vi "Get Required Driver Type.vi"(8 "error in (no error)":errorcluster, 11 "DMM Msg in":refnum<class "DMM Msg.lvclass">) -> (0 "error out":errorcluster, 2 "Required Driver Type":refnum<class "Instrument Driver.lvclass">, 3 "DMM Msg out":refnum<class "DMM Msg.lvclass">)   [LabVIEW 2020, in "DMM Msg.lvlib" / "DMM Msg.lvclass"]
doc: "Get the Required Driver Type for execution of the Instrument Msg."
uses:
  DMM Msg.lvclass
  PPL/HDH.Actor Framework.Core.Instrument Driver.lvlibp/Instrument Driver/Instrument Driver.lvclass
  PPL/HDH.Driver.DMM.lvlibp/DMM Driver.lvclass
  C:/Current projects/WS/PPL/HDH.Actor Framework.Core.Instrument Driver.lvlibp/Instrument Driver/Instrument Driver.lvclass
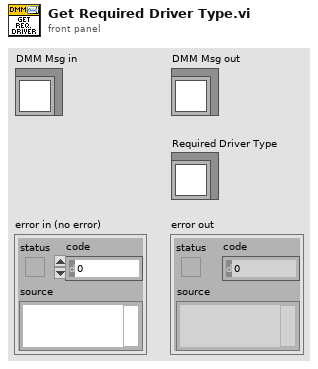
[diagram p1: front panel]
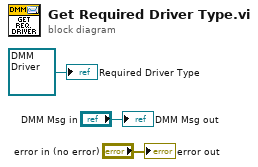
[diagram p0: block diagram]
diagram:
  "error out" <- "error in (no error)"
  "DMM Msg out" <- "DMM Msg in"
  "Required Driver Type" <- refnum<class "DMM Driver.lvclass"> refnum ("HDH.Driver.DMM.lvlibp:DMM Driver.lvclass")
